vi "LED Lights Set Color.vi"(6 "error in":errorcluster, 7 "LED Lights Ref In":T1={"I2CDevRef"={"DevStatus"={"status"=FALSE, "code"=0, "source"=""}, "Device Address"=0, "Handle"=0, "I2C Bus"=enum."Invalid"}} {"I2CDevRef"."Device Address" format="%.0x"}, 10 "Color":cluster{"Red":dbl, "Green":dbl, "Blue":dbl}, 11 "Light ID":u8) -> (0 "error out":errorcluster, 3 "LED Lights Ref Out":T1={"I2CDevRef"={"DevStatus"={"status"=FALSE, "code"=0, "source"=""}, "Device Address"=0, "Handle"=0, "I2C Bus"=enum."Invalid"}} {"I2CDevRef"."Device Address" format="%.0x"})   [LabVIEW 2015]
uses:
  LED Lights Ref.ctl
  <vilib>/Rock Robotics/WPI/I2C/WPI_I2CDevRef.ctl
  <vilib>/Rock Robotics/SystemInterfaces/i2clib/i2c_bus.ctl
  <vilib>/Rock Robotics/Network Tables/NT Write Boolean.vi
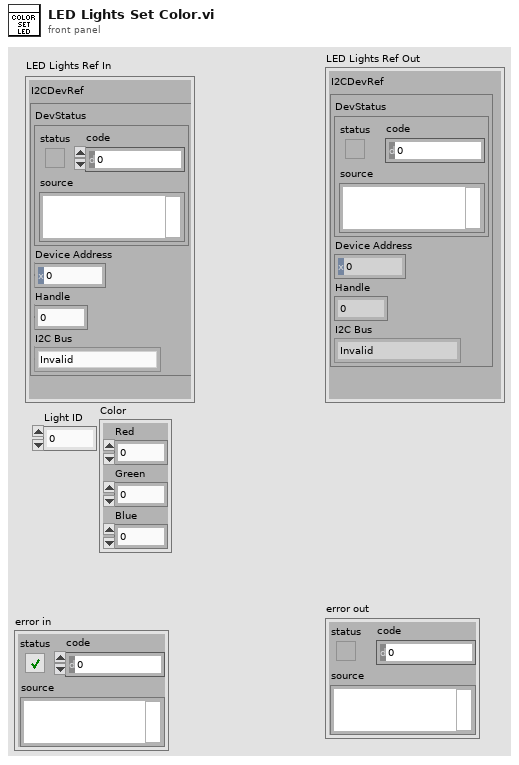
[diagram p1: front panel]
types:
  T1 = typedef "LED Lights Ref.ctl" = cluster{"I2CDevRef":T2}
  T2 = typedef "WPI_I2CDevRef.ctl" = cluster{"DevStatus":errorcluster, "Device Address":u8, "Handle":i32, "I2C Bus":T3}
  T3 = typedef "i2c_bus.ctl" = enum16{"I2C On-Board", "I2C MXP", "Invalid"}
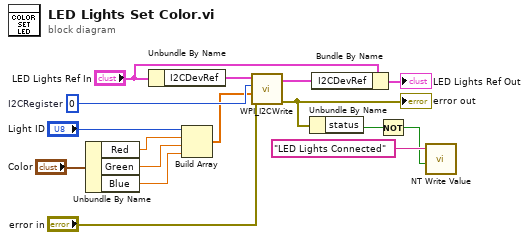
[diagram p0: block diagram]
diagram:
  w15 = u8 0  # I2CRegister
  n1 = Unbundle By Name("Color") -> ("Red"=w3:dbl, "Green"=w2:dbl, "Blue"=w1:dbl)
  n2 = Unbundle By Name("LED Lights Ref In") -> ("I2CDevRef"=w16:T2)
  n3 = Build Array("Light ID", w3, w2, w1) -> (w13:dbl[])
  n4 = call <vilib>:"WPI_I2CWrite.vi"("error in (no error)"="error in", "I2CDataToSend"=w13, "I2CRegister"=w15, "I2CDevRef"=w16) -> ("error out"=w8:errorcluster, "I2CDevRef"=w11:T2)  [unwired: 6 in]
  "error out" <- w8
  n5 = Unbundle By Name(w8) -> ("status"=w6:bool)
  n6 = Bundle By Name(cluster="LED Lights Ref In", "I2CDevRef"=w11) -> (→"LED Lights Ref Out":T1)
  n7 = Not(x=w6) -> (.not. x?=w5:bool)
  n8 = call-poly <vilib>:"NT Write Value.vi"("Boolean"=w5, "Name"="LED Lights Connected") -> ()  [unwired: 9 in, 1 out]
